vi "Drive space error handler.vi"(8 "error in (no error)":errorcluster, 10 "Saves folder path":path, 11 "String in":string) -> (2 "Boolean":bool, 3 "String out":string)   [LabVIEW 2020]
uses:
  Global Variables/General Globals.vi
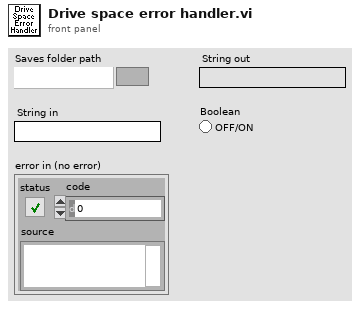
[diagram p1: front panel]
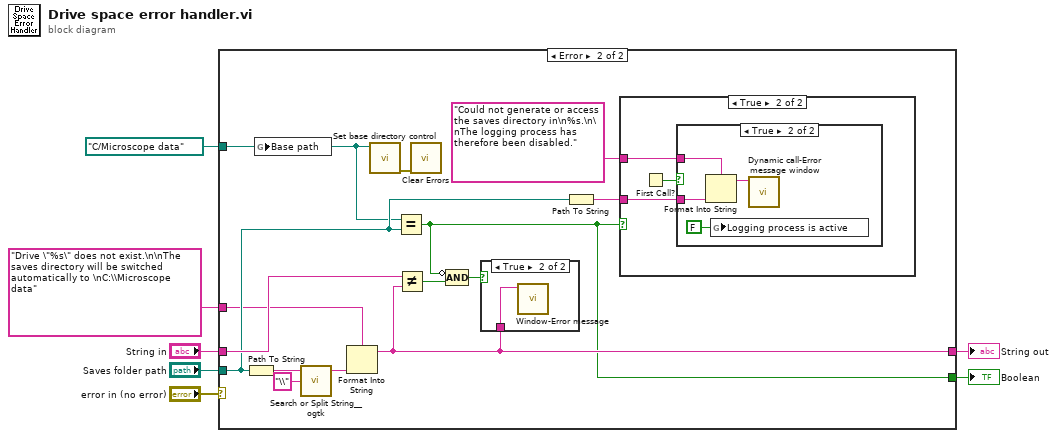
[diagram p0: block diagram]
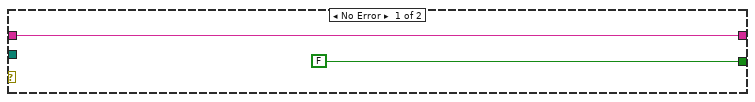
[diagram p2: hidden frame]
diagram:
  n1 = case shown="Error" "error in (no error)" {
    tunnel: "Saves folder path" -> [_ w18]
    tunnel: [w9 w22] -> w3
    tunnel: "String in" -> [w9 w23]
    tunnel: [FALSE w13] -> w5
    tunnel: "Drive \"%s\" does not exist.\n\nThe saves directory will be switched automatically to \nC:\\Microscope data" ("Error Source") -> [_ w12]
    tunnel: path "C:/Microscope data" ("Base path") -> [_ w10]
    frame No Error {
    }
    frame Error {
      n2 = Path To String(path=w18) -> (string=w20:string)
      n3 = global write "General Globals.vi" "Base path"(w10) -> ()
      n4 = call <userlib>:"Search or Split String__ogtk.vi"("search string/char (-)"="\\", "string"=w20) -> ("substring before match"=w19:string)  [unwired: 1 in, 2 out]
      n5 = Format Into String(format string=w12, w19) -> (resulting string=w22:string)  [unwired: 2 in, 1 out]
      n6 = call "Set base directory control.vi"("Base path"=w10) -> ("error out"=w11:errorcluster)  [unwired: 10 in]
      n7 = Equal?(x=w10, y=w18) -> (x = y?=w13:bool)
      n8 = Not Equal?(x=w23, y=w22) -> (x != y?=w15:bool)
      n9 = call <vilib>:"Clear Errors.vi"("error in (no error)"=w11) -> ()  [unwired: 5 in, 2 out]
      n10 = Compound Arithmetic op=AND(invert w13, w15) -> (w16:bool)
      n11 = case shown="True" w16 {
        tunnel: w22 -> [_ w31]
        frame False {
        }
        frame True {
          n12 = call "Window-Error message.vi"("Message"=w31) -> ()  [unwired: 10 in, 1 out]
        }
      }
      n13 = Path To String(path=w18) -> (string=w17:string)
      n14 = case shown="True" w13 {
        tunnel: "Could not generate or access the saves directory in\n%s.\n\nThe logging process has therefore been disabled." ("Error Source") -> [_ w26]
        tunnel: w17 -> [_ w25]
        frame False {
        }
        frame True {
          n15 = First Call?() -> (First Call?: T/F=w24:bool)
          n16 = case shown="True" w24 {
            tunnel: w26 -> [_ w30]
            tunnel: w25 -> [_ w29]
            frame False {
            }
            frame True {
              n17 = Format Into String(format string=w30, w29) -> (resulting string=w28:string)  [unwired: 2 in, 1 out]
              n18 = global write "General Globals.vi" "Logging process is active"(FALSE ("Logging process is active")) -> ()
              n19 = call "Dynamic call-Error message window.vi"("Error Message"=w28) -> ()  [unwired: 10 in, 1 out]
            }
          }
        }
      }
    }
  }
  "Boolean" <- w5
  "String out" <- w3
